vi "Send Graphite Metric.vi"(8 "error in (no error)":errorcluster, 10 "Cluster":cluster{"metric":string, "value":dbl}, 11 "TCP Network Connection in":refnum<k5>) -> (0 "error out":errorcluster, 1 "status":bool, 2 "Message":string="graphite", 3 "TCP Network Connection out":refnum<k5>)   [LabVIEW 2023]
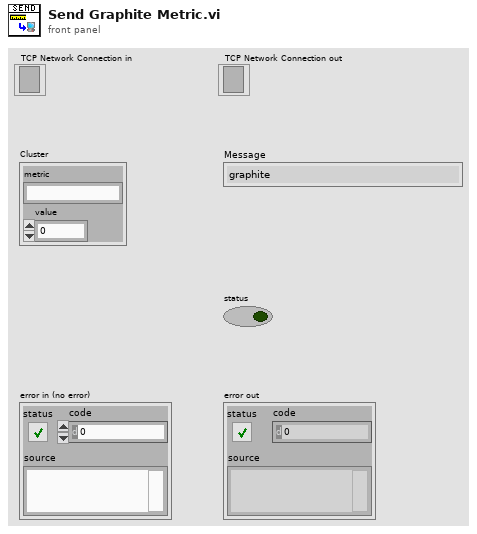
[diagram p1: front panel]
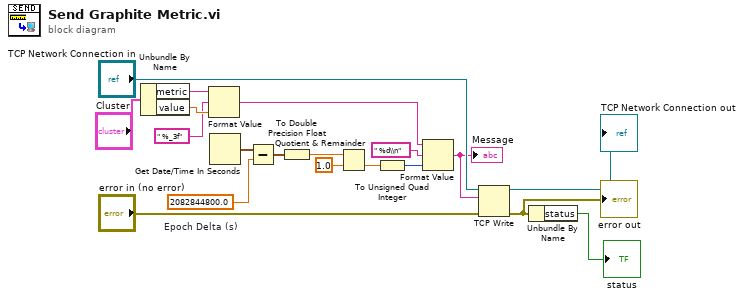
[diagram p0: block diagram]
diagram:
  w6 = 2082844800.0  # Epoch Delta (s)
  n1 = Unbundle By Name("Cluster") -> ("metric"=w18:string, "value"=w17:dbl)
  n2 = Format Value(string ("")=w18, format string=" %_3f" ("Message"), value (0)=w17) -> (output string=w7:string)
  n3 = Get Date/Time In Seconds() -> (seconds since 1Jan1904=w5:timestamp)
  n4 = Subtract(x=w5, y=w6) -> (x-y=w4:timestamp)
  n5 = To Double Precision Float(number=w4) -> (double precision float=w3:dbl)
  n6 = Quotient & Remainder(x=w3, y=1.0) -> (floor(x/y)=w1:dbl)  [unwired: 1 out]
  n7 = To Unsigned Quad Integer(1:w1) -> (0:w9:u64)
  n8 = Format Value(string ("")=w7, format string=" %d\\n" ("Message"), value (0)=w9) -> (output string=w11:string)
  "Message" <- w11
  n9 = TCP Write(connection ID="TCP Network Connection in", data in=w11, error in (no error)="error in (no error)") -> (connection ID out=→"TCP Network Connection out":refnum<k5>, error out=w15:errorcluster)  [unwired: 1 in, 1 out]
  "error out" <- w15
  n10 = Unbundle By Name(w15) -> ("status"=→"status":bool)
